vi "simulation.vi"() -> ()   [LabVIEW 2024]
uses:
  <vilib>/Analysis/baseanly.llb/Mean (DBL).vi
  <vilib>/Utility/file.llb/Read Delimited Spreadsheet (DBL).vi
  <vilib>/Analysis/NI_AALBase.lvlib
panel:
  out "XY Graph 7":cluster{dbl[], dbl[]}[](graph)
  out "XY Graph 6":cluster{dbl[], dbl[]}[](graph)
  out "XY Graph 5":cluster{dbl[], dbl[]}[](graph)
  out "XY Graph 4":cluster{dbl[], dbl[]}[](graph)
  out "XY Graph 3":cluster{dbl[], sgl[]}[](graph)
  out "XY Graph 2":cluster{dbl[], dbl[]}[](graph)
  out "period(Hz)":dbl(knob) scale=0.0..40.0
  out "Histogram Graph":cluster{i32[], u32[]}(graph)
  out "time":dbl
  out "Slide":dbl(slide) scale=0.0..100.0
  out "error out":errorcluster
  in  "stop":bool
  in  "file path (dialog if empty)":path
  out "XY Graph":cluster{dbl[], dbl[]}(graph)
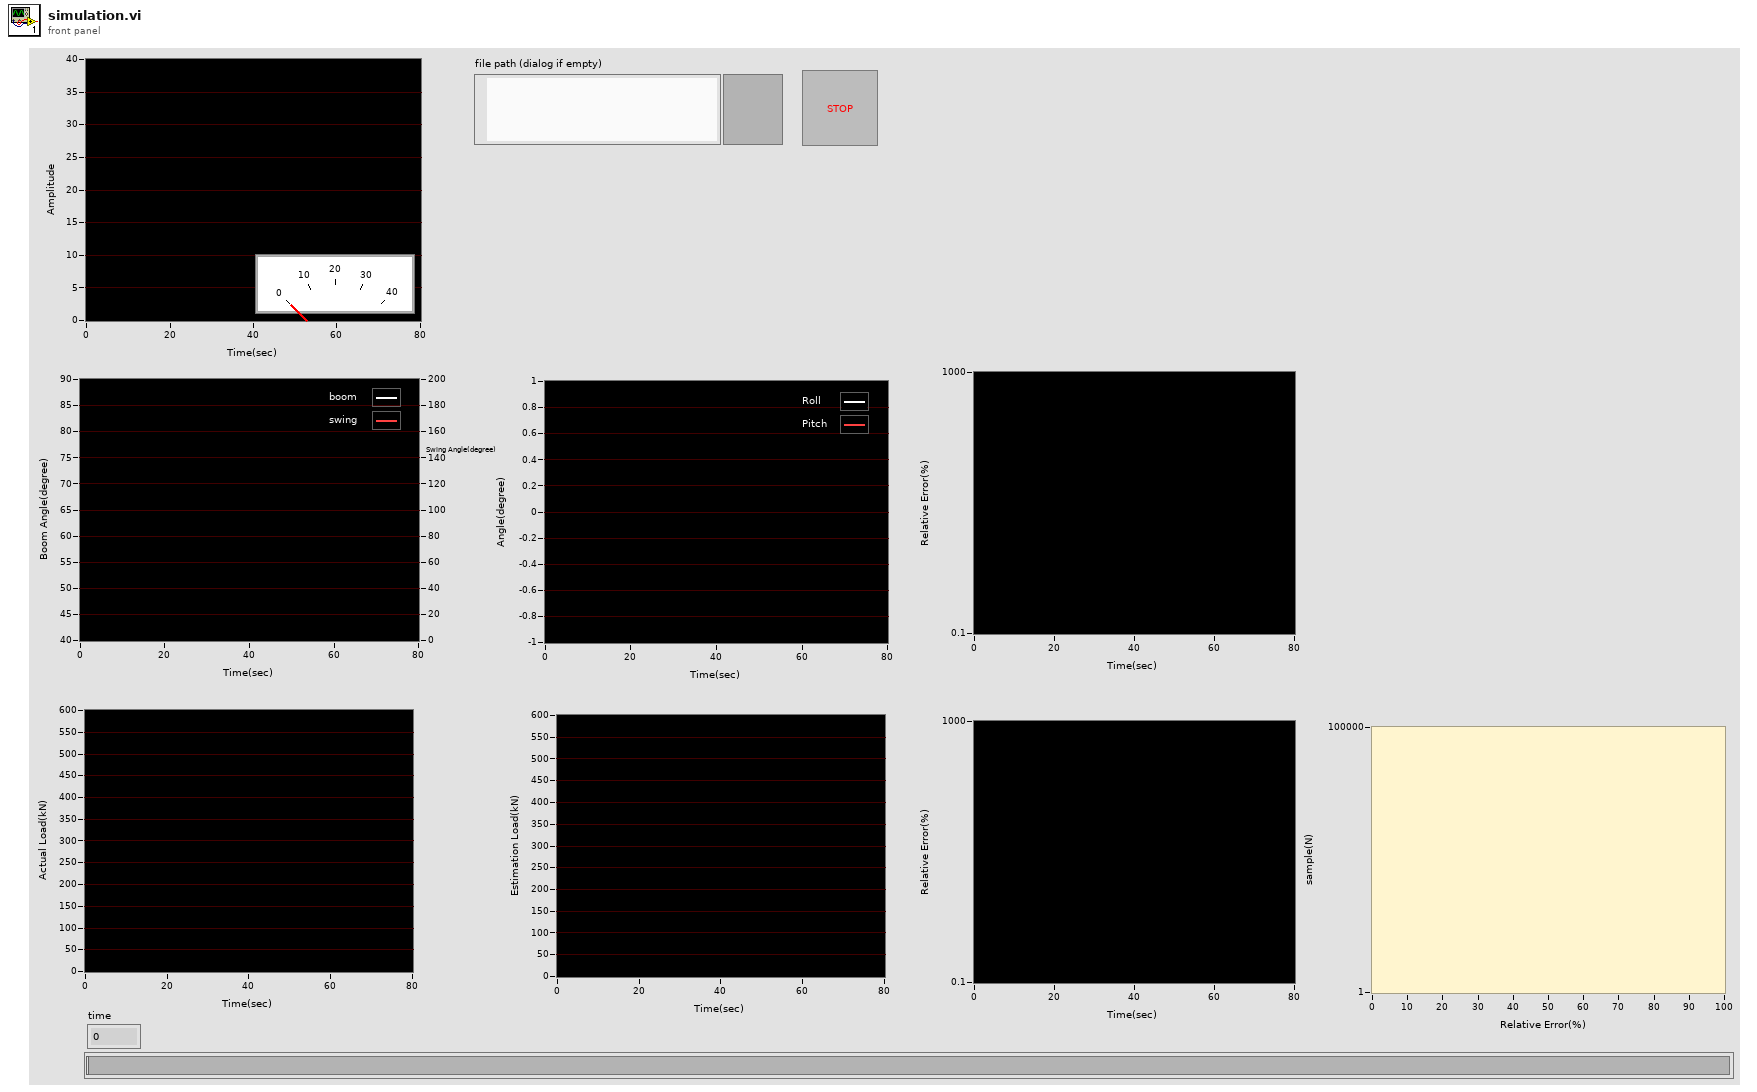
[diagram p1: front panel]
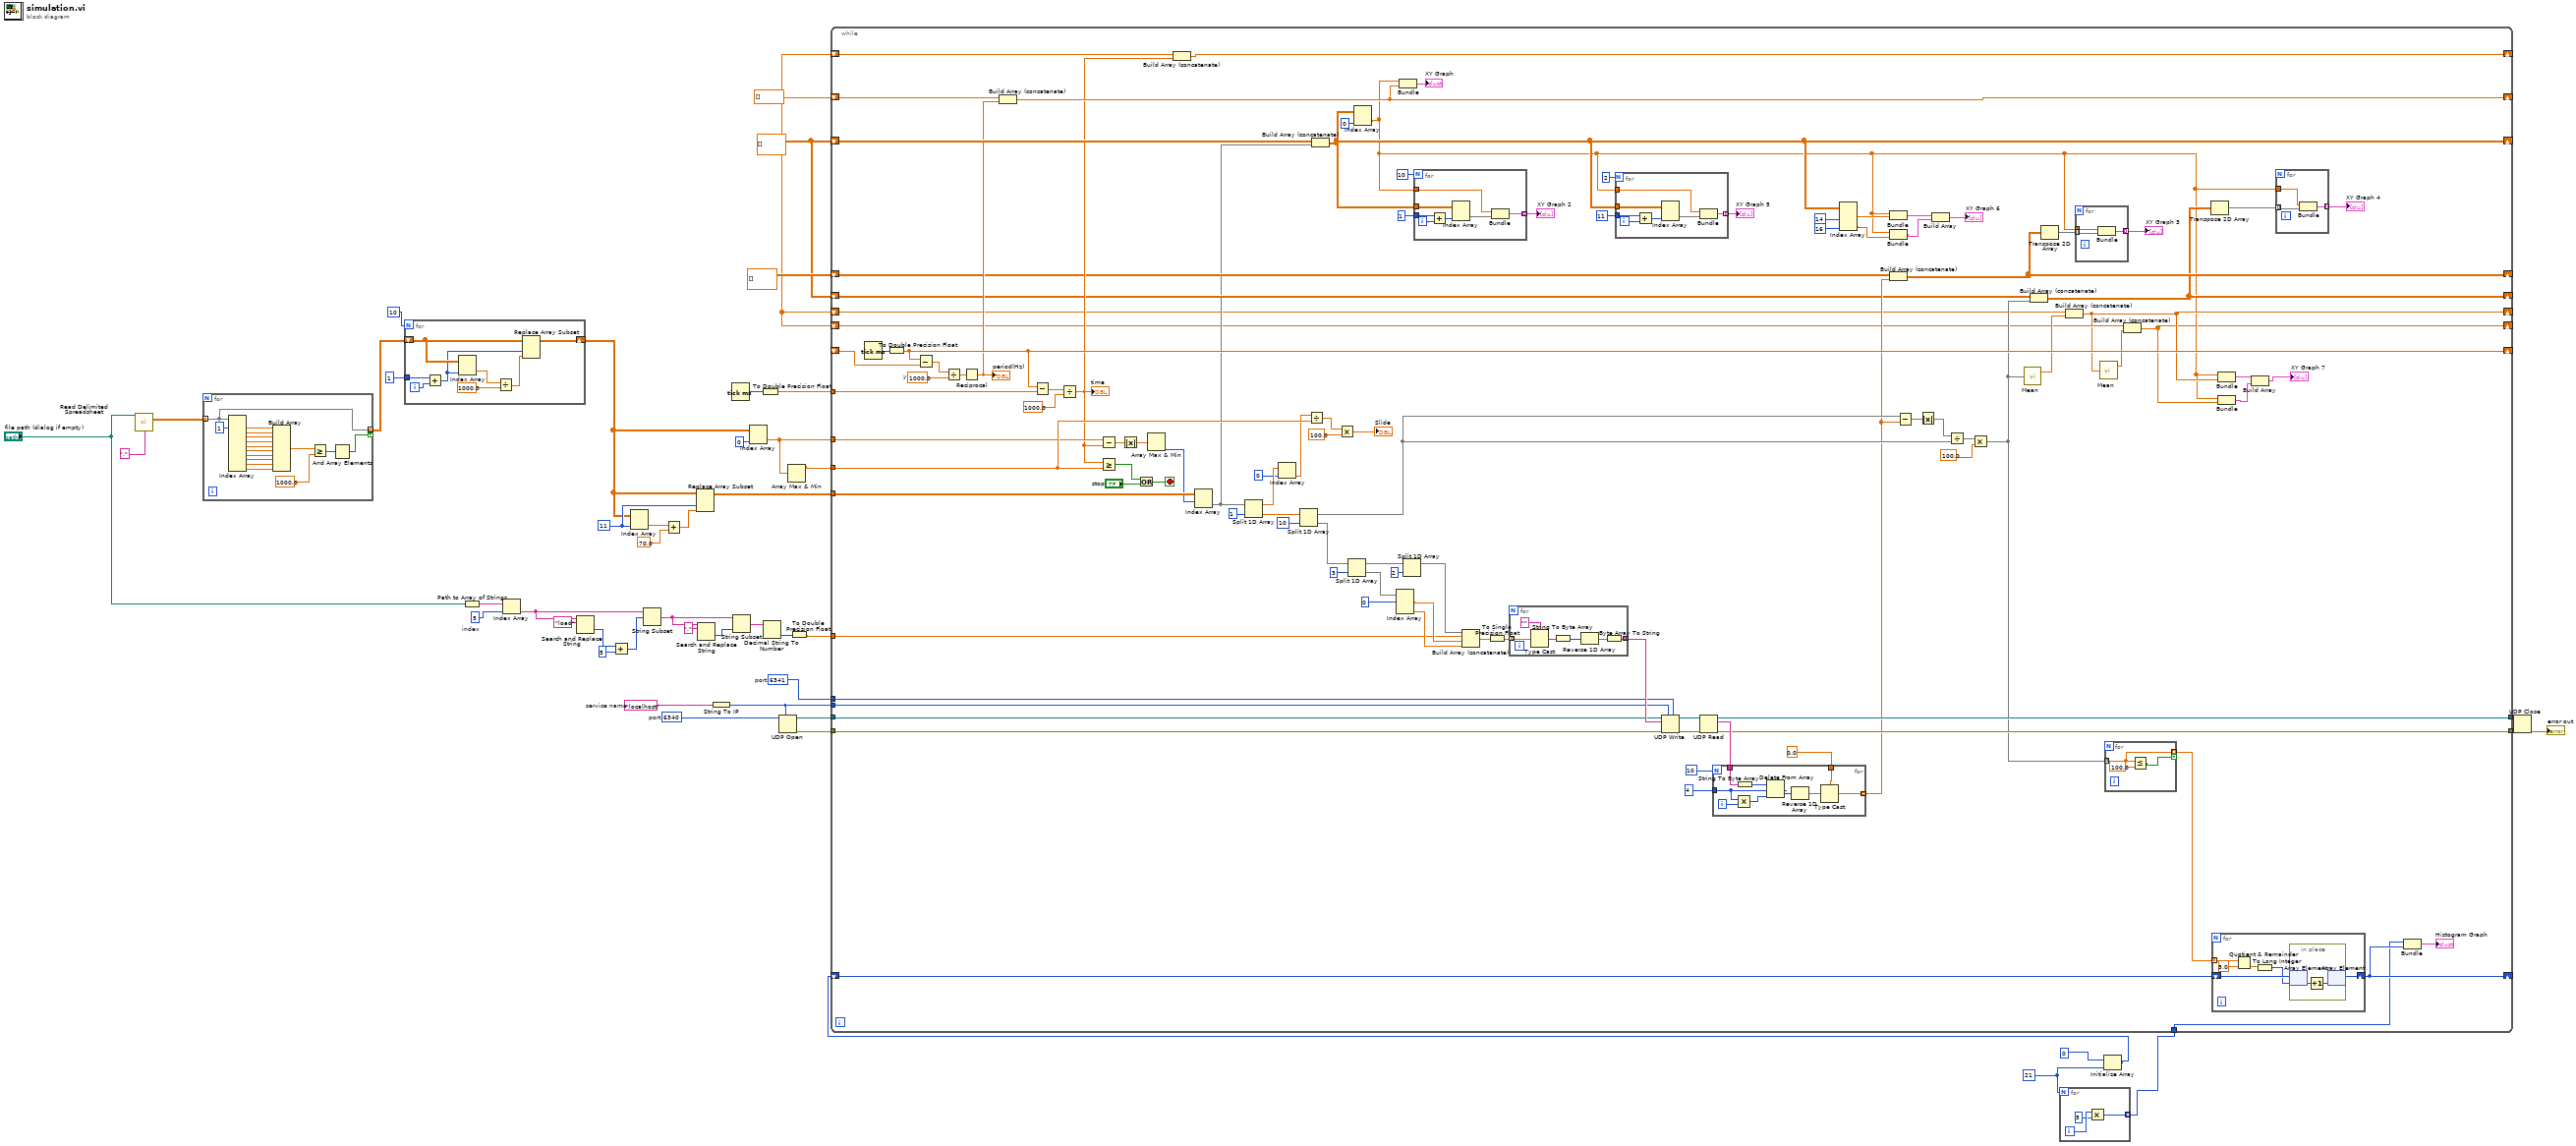
[diagram p0: block diagram]
diagram:
  w6 = 11 ("disabled index (col)")
  w11 = dbl[][] []
  w1 = dbl[] []
  w27 = 21
  w29 = 5  # index
  w38 = u16 6341  # port
  w40 = "localhost"  # service name
  w39 = u16 6340  # port
  n1 = call-poly <vilib>:"Read Delimited Spreadsheet.vi"("file path (dialog if empty)"="file path (dialog if empty)", "delimiter (\\t)"="," ("delimiter (\\t)")) -> ("all rows"=w28:dbl[][])  [unwired: 8 in, 5 out]
  n2 = for {
    tunnel: w28 -> [w48] mode=indexing
    tunnel: [w48] -> w3 mode=indexing if=w47
    n3 = Index Array(array=w48, index #1=1 ("index")) -> (element #1=w61:dbl, element #2=w60:dbl, element #3=w59:dbl, element #4=w58:dbl, element #5=w57:dbl, element #6=w56:dbl, element #7=w55:dbl, element #8=w54:dbl, element #9=w53:dbl, element #10=w52:dbl)  [unwired: 9 in]
    n4 = Build Array(w61, w60, w59, w58, w57, w56, w55, w54, w53, w52) -> (w50:dbl[])
    n5 = Greater Or Equal?(x=w50, y=1000.0) -> (x >= y?=w49:bool[])
    n6 = And Array Elements(Boolean array=w49) -> (logical AND=w47:bool)
  }
  n7 = for {
    N: 10 -> [_]
    tunnel: 1 -> [w70]
    shift-right: [w67] -> w2
    shift-left: w3 -> [w66]
    i -> [w69]
    n8 = Add(x=w70, y=w69) -> (x+y=w63:i32)
    n9 = Index Array(array=w66, index (col)=w63) -> (element=w65:dbl[])  [unwired: 1 in]
    n10 = Divide(x=w65, y=1000.0) -> (x/y=w64:dbl[])
    n11 = Replace Array Subset "Replace Array Subset"(array=w66, new element=w64, index (col)=w63) -> (w67:dbl[][])  [unwired: 1 in]
  }
  n12 = Path to Array of Strings(0:"file path (dialog if empty)") -> (2:w30:string[])  [unwired: 1 out]
  n13 = Index Array(array=w30, index=w29) -> (element=w14:string)
  n14 = Search and Replace String(input string=w14, search string="load") -> (offset past replacement=w18:i32)  [unwired: 6 in, 3 out]
  n15 = Add(x=w18, y=5) -> (x+y=w19:i32)
  n16 = Index Array(array=w2, index (col)=w6) -> (element=w9:dbl[])  [unwired: 1 in]
  n17 = String Subset(string=w14, offset (0)=w19) -> (substring=w21:string)  [unwired: 1 in]
  n18 = Add(x=w9, y=70.0) -> (x+y=w7:dbl[])
  n19 = Replace Array Subset "Replace Array Subset"(array=w2, new element=w7, index (col)=w6) -> (w10:dbl[][])  [unwired: 1 in]
  n20 = Search and Replace String(input string=w21, search string=".") -> (offset past replacement=w20:i32)  [unwired: 6 in, 3 out]
  n21 = String To IP(1:w40) -> (0:w35:u32)
  n22 = Tick Count (ms)() -> (millisecond timer value=w45:u32)
  n23 = String Subset(string=w21, length (rest)=w20) -> (substring=w22:string)  [unwired: 1 in]
  n24 = Index Array "Index Array"(array=w2, index (col)=0 ("disabled index (col)")) -> (element=w42:dbl[])  [unwired: 1 in]
  n25 = To Double Precision Float(number=w45) -> (double precision float=w44:dbl)
  n26 = Decimal String To Number(string=w22) -> (number=w23:i32)  [unwired: 2 in, 1 out]
  n27 = UDP Open(7:w35, 11:w39) -> (port=w37:refnum<k16>, 0:w36:errorcluster)  [unwired: 3 in, 1 out]
  n28 = Array Max & Min(array=w42) -> (max value=w41:dbl)  [unwired: 3 out]
  n29 = To Double Precision Float(number=w23) -> (double precision float=w13:dbl)
  n30 = for {
    N: w27 -> [_]
    tunnel: [w71] -> w24 mode=indexing
    i -> [w73]
    n31 = Multiply(x=w73, y=5) -> (x*y=w71:i32)
  }
  n32 = Initialize Array(u32 0 ("y"), w27) -> (w25:u32[])
  n33 = while {
    tunnel: w44 -> [w178]
    tunnel: w10 -> [w173]
    tunnel: w42 -> [w119]
    tunnel: w41 -> [w134]
    tunnel: w38 -> [w158]
    tunnel: w37 -> [w157]
    tunnel: w36 -> [w156]
    tunnel: w35 -> [w155]
    tunnel: [w148] -> w33
    tunnel: [w147] -> w32
    shift-right: [w143] -> _
    shift-left: _ -> [w142]
    shift-right: [w125] -> _
    shift-left: w25 -> [w126]
    tunnel: w24 -> [w124]
    shift-right: [w115] -> _
    shift-left: w1 -> [w122]
    tunnel: w13 -> [w121]
    shift-right: [w92] -> _
    shift-left: w11 -> [w120]
    shift-right: [w112] -> _
    shift-left: w1 -> [w114]
    shift-right: [w106] -> _
    shift-left: sgl[][] [] -> [w108]
    shift-right: [w82] -> _
    shift-left: w11 -> [w103]
    shift-right: [w80] -> _
    shift-left: w1 -> [w84]
    shift-right: [w77] -> _
    shift-left: w1 -> [w81]
    stop <- w168 stop-if-true
    w145 = 1000.0  # y
    n34 = Tick Count (ms)() -> (millisecond timer value=w179:u32)
    n35 = To Double Precision Float(number=w179) -> (double precision float=w143:dbl)
    n36 = Subtract(x=w143, y=w142) -> (x-y=w146:dbl)
    n37 = Divide(x=w146, y=w145) -> (x/y=w144:dbl)
    n38 = Reciprocal(x=w144) -> (1/x=w116:dbl)
    "period(Hz)" <- w116
    n39 = Build Array (concatenate)(w122, w116) -> (w115:dbl[])
    n40 = Subtract(x=w143, y=w178) -> (x-y=w177:dbl)
    n41 = Divide(x=w177, y=1000.0) -> (x/y=w113:dbl)
    "time" <- w113
    n42 = Subtract(x=w119, y=w113) -> (x-y=w175:dbl[])
    n43 = Greater Or Equal?(x=w113, y=w134) -> (x >= y?=w169:bool)
    n44 = Absolute Value(x=w175) -> (abs(x)=w174:dbl[])
    n45 = Or(x=w169, y="stop") -> (x .or. y?=w168:bool)
    n46 = Array Max & Min(array=w174) -> (min index (indices)=w172:i32)  [unwired: 3 out]
    n47 = Build Array (concatenate)(w114, w113) -> (w112:dbl[])
    n48 = Index Array "Index Array"(array=w173, index (row)=w172) -> (element=w93:dbl[])  [unwired: 1 in]
    n49 = Split 1D Array(array=w93, index=1) -> (first subarray=w133:dbl[], second subarray=w166:dbl[])
    n50 = Index Array(array=w133, index=0) -> (element=w131:dbl)
    n51 = Split 1D Array(array=w166, index=10) -> (first subarray=w163:dbl[], second subarray=w164:dbl[])
    n52 = Divide(x=w131, y=w134) -> (x/y=w130:dbl)
    n53 = Build Array (concatenate)(w120, w93) -> (w92:dbl[][])
    n54 = Multiply(x=w130, y=100.0) -> (x*y=→"Slide":dbl)
    n55 = Split 1D Array(array=w164, index=3) -> (first subarray=w96:dbl[], second subarray=w162:dbl[])
    n56 = Index Array(array=w92, index (col)=0 ("disabled index (col)")) -> (element=w78:dbl[])  [unwired: 1 in]
    n57 = Index Array(array=w162, index #1=0 ("index")) -> (element #1=w141:dbl, element #3=w140:dbl)  [unwired: 2 in, 1 out]
    n58 = Bundle(w78, w115) -> (→"XY Graph":cluster{dbl[], dbl[]})  [unwired: 1 in]
    n59 = Split 1D Array(array=w96, index=2) -> (first subarray=w94:dbl[])  [unwired: 1 out]
    n60 = for {
      N: 10 -> [_]
      tunnel: w92 -> [w199]
      tunnel: w78 -> [w198]
      tunnel: 1 -> [w197]
      tunnel: [w194] -> w109 mode=indexing
      i -> [w196]
      n61 = Add(x=w197, y=w196) -> (x+y=w195:i32)
      n62 = Index Array(array=w199, index (col)=w195) -> (element=w193:dbl[])  [unwired: 1 in]
      n63 = Bundle(w198, w193) -> (w194:cluster{dbl[], dbl[]})  [unwired: 1 in]
    }
    "XY Graph 2" <- w109
    n64 = Build Array (concatenate)(w94, w121, w141, w140) -> (w160:dbl[])
    n65 = To Single Precision Float(number=w160) -> (single precision float=w139:sgl[])
    n66 = for {
      tunnel: w139 -> [w225] mode=indexing
      tunnel: [w220] -> w159 mode=concatenating
      n67 = Type Cast(type="" ("data out"), x=w225) -> (*(type *) &x=w223:string)
      n68 = String To Byte Array(string=w223) -> (unsigned byte array=w222:u8[])
      n69 = Reverse 1D Array(array=w222) -> (reversed array=w221:u8[])
      n70 = Byte Array To String(unsigned byte array=w221) -> (string=w220:string)
    }
    n71 = for {
      N: 2 -> [_]
      tunnel: w92 -> [w186]
      tunnel: w78 -> [w185]
      tunnel: 11 -> [w184]
      tunnel: [w181] -> w98 mode=indexing
      i -> [w183]
      n72 = Add(x=w184, y=w183) -> (x+y=w182:i32)
      n73 = Index Array(array=w186, index (col)=w182) -> (element=w180:dbl[])  [unwired: 1 in]
      n74 = Bundle(w185, w180) -> (w181:cluster{dbl[], dbl[]})  [unwired: 1 in]
    }
    "XY Graph 5" <- w98
    n75 = UDP Write(address=w155, port or service name=w158, connection ID=w157, data in=w159, 8:w156) -> (error out=w150:errorcluster, 3:w151:refnum<k16>)  [unwired: 1 in]
    n76 = UDP Read(connection ID=w151, 8:w150) -> (data out=w149:string, error out=w147:errorcluster, 3:w148:refnum<k16>)  [unwired: 2 in, 2 out]
    n77 = for {
      N: 10 -> [_]
      tunnel: w149 -> [w219]
      tunnel: 4 ("length") -> [w216]
      tunnel: sgl 0.0 -> [w212]
      tunnel: [w211] -> w107 mode=indexing
      i -> [w217]
      n78 = Multiply(x=w216, y=w217) -> (x*y=w215:i32)
      n79 = String To Byte Array(string=w219) -> (unsigned byte array=w218:u8[])
      n80 = Delete From Array(array=w218, length=w216, index=w215) -> (deleted portion=w214:u8[])  [unwired: 1 out]
      n81 = Reverse 1D Array(array=w214) -> (reversed array=w213:u8[])
      n82 = Type Cast(type=w212, x=w213) -> (*(type *) &x=w211:sgl)
    }
    n83 = Index Array(array=w92, index (col) #1=14 ("disabled index (col)"), index (col) #2=16 ("disabled index (col)")) -> (element #1=w88:dbl[], element #2=w87:dbl[])  [unwired: 2 in]
    n84 = Bundle(w78, w88) -> (w91:cluster{dbl[], dbl[]})  [unwired: 1 in]
    n85 = Bundle(w78, w87) -> (w90:cluster{dbl[], dbl[]})  [unwired: 1 in]
    n86 = Build Array (concatenate)(w108, w107) -> (w106:sgl[][])
    n87 = Subtract(x=w163, y=w107) -> (x-y=w138:dbl[])
    n88 = Absolute Value(x=w138) -> (abs(x)=w137:dbl[])
    n89 = Build Array(w91, w90) -> (→"XY Graph 6":cluster{dbl[], dbl[]}[])
    n90 = Divide(x=w137, y=w163) -> (x/y=w136:dbl[])
    n91 = Multiply(x=w136, y=100.0) -> (x*y=w102:dbl[])
    n92 = call-poly <vilib>:"Mean.vi"("X"=w102) -> ("mean"=w83:dbl)  [unwired: 1 out]
    n93 = Build Array (concatenate)(w103, w102) -> (w82:dbl[][])
    n94 = Transpose 2D Array(2D array=w106) -> (transposed array=w105:sgl[][])
    n95 = Build Array (concatenate)(w84, w83) -> (w80:dbl[])
    n96 = for {
      tunnel: w78 -> [w192]
      tunnel: [w191] -> w104 mode=indexing
      tunnel: w105 -> [w190] mode=indexing
      n97 = Bundle(w192, w190) -> (w191:cluster{dbl[], sgl[]})  [unwired: 1 in]
    }
    "XY Graph 3" <- w104
    n98 = call-poly <vilib>:"Mean.vi"("X"=w80) -> ("mean"=w79:dbl)  [unwired: 1 out]
    n99 = for {
      tunnel: w102 -> [w209] mode=indexing
      tunnel: [w209] -> w123 mode=indexing if=w208
      n100 = Less Or Equal?(x=w209, y=100.0) -> (x <= y?=w208:bool)
    }
    n101 = Build Array (concatenate)(w81, w79) -> (w77:dbl[])
    n102 = Transpose 2D Array(2D array=w82) -> (transposed array=w100:dbl[][])
    n103 = for {
      tunnel: w123 -> [w202] mode=indexing
      shift-right: [w204] -> w125
      shift-left: w126 -> [w205]
      n104 = Quotient & Remainder(x=w202, y=5.0) -> (floor(x/y)=w201:dbl)  [unwired: 1 out]
      n105 = To Long Integer(number=w201) -> (32bit integer=w200:i32)
      n106 = in-place {
        n107 = in-place-array #1(w205, w200) -> (w207:u32)
        n108 = Increment(x=w207) -> (x+1=w206:u32)
        n109 = in-place-array #1(w206) -> (w204:u32[])  [unwired: 1 out]
      }
    }
    n110 = Bundle(w78, w80) -> (w76:cluster{dbl[], dbl[]})  [unwired: 1 in]
    n111 = Bundle(w78, w77) -> (w75:cluster{dbl[], dbl[]})  [unwired: 1 in]
    n112 = Build Array(w76, w75) -> (→"XY Graph 7":cluster{dbl[], dbl[]}[])
    n113 = for {
      tunnel: w78 -> [w189]
      tunnel: [w188] -> w101 mode=indexing
      tunnel: w100 -> [w187] mode=indexing
      n114 = Bundle(w189, w187) -> (w188:cluster{dbl[], dbl[]})  [unwired: 1 in]
    }
    "XY Graph 4" <- w101
    n115 = Bundle(w124, w125) -> (→"Histogram Graph":cluster{i32[], u32[]})  [unwired: 1 in]
  }
  n116 = UDP Close(connection ID=w33, 8:w32) -> (error out=→"error out":errorcluster)  [unwired: 1 out]
